vi "AlliGator Get Python Plugin API Version.vi"(8 "error in (no error)":errorcluster, 10 "Source":string, 11 "Script Header":string) -> (0 "error out":errorcluster, 1 "API Version":string, 3 "Script Header - Version":string)   [LabVIEW 2021, in "AlliGator Python Plugins.lvlib"]
uses:
  AlliGator Python Plugins.lvlib
panel:
  # "see the AlliGator License on the block diagram (Ctrl+E or Window:Show Block Diagram)"
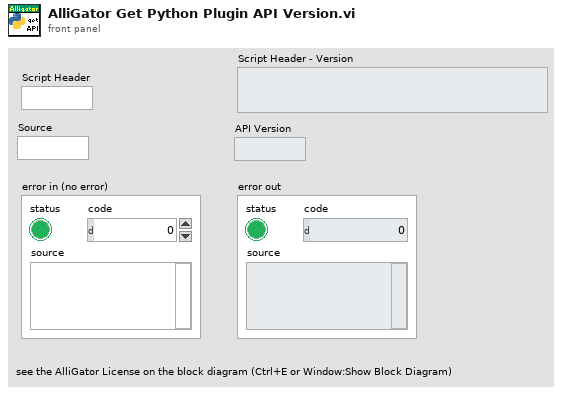
[diagram p1: front panel]
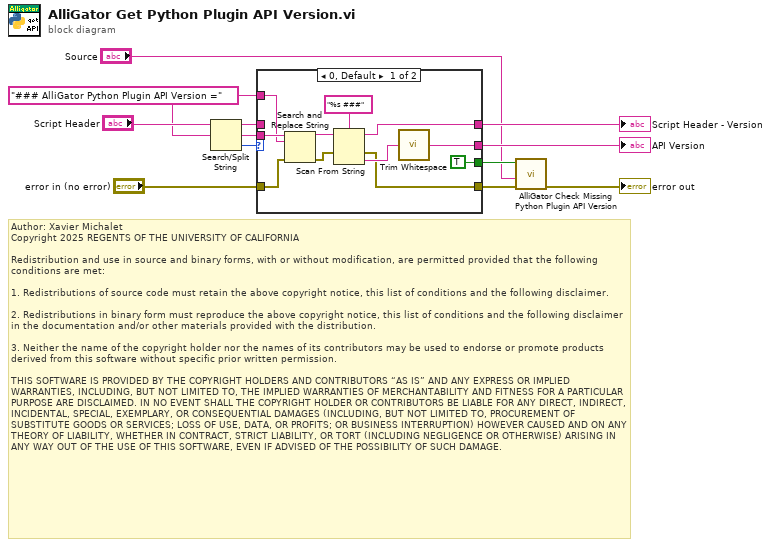
[diagram p0: block diagram]
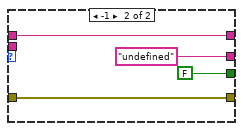
[diagram p2: hidden frame]
diagram:
  w9 = "### AlliGator Python Plugin API Version =" ("operators (none)")
  # "Author: Xavier Michalet\nCopyright 2025 REGENTS OF THE UNIVERSITY OF CALIFORNIA\n\nRedistribution and use in source and binary forms, with or without modification, are permitted provided that the following conditions are met:\n\n1. Redistributions of source code must retain the above copyright notice, this list of conditions and the following disclaimer.\n\n2. Redistributions in binary form must reproduce the above copyright notice, this list of conditions and the following disclaimer in the documentation and/or other materials provided with the distribution.\n\n3. Neither the name of the copyright holder nor the names of its contributors may be used to endorse or promote products derived from this software without specific prior written permission.\n\nTHIS SOFTWARE IS PROVIDED BY THE COPYRIGHT HOLDERS AND CONTRIBUTORS “AS IS” AND ANY EXPRESS OR IMPLIED WARRANTIES, INCLUDING, BUT NOT LIMITED TO, THE IMPLIED WARRANTIES OF MERCHANTABILITY AND FITNESS FOR A PARTICULAR PURPOSE ARE DISCLAIMED. IN NO EVENT SHALL THE COPYRIGHT HOLDER OR CONTRIBUTORS BE LIABLE FOR ANY DIRECT, INDIRECT, INCIDENTAL, SPECIAL, EXEMPLARY, OR CONSEQUENTIAL DAMAGES (INCLUDING, BUT NOT LIMITED TO, PROCUREMENT OF SUBSTITUTE GOODS OR SERVICES; LOSS OF USE, DATA, OR PROFITS; OR BUSINESS INTERRUPTION) HOWEVER CAUSED AND ON ANY THEORY OF LIABILITY, WHETHER IN CONTRACT, STRICT LIABILITY, OR TORT (INCLUDING NEGLIGENCE OR OTHERWISE) ARISING IN ANY WAY OUT OF THE USE OF THIS SOFTWARE, EVEN IF ADVISED OF THE POSSIBILITY OF SUCH DAMAGE."
  n1 = Search/Split String(string="Script Header", search string/char (-)=w9) -> (substring before match=w6:string, match + rest of string=w10:string, offset of match=w11:i32)  [unwired: 1 in]
  n2 = case shown="0, Default" w11 {
    tunnel: w10 -> [w23 _]
    tunnel: w9 -> [w22 _]
    tunnel: [w13 w26] -> w8
    tunnel: "error in (no error)" -> [w19 w27]
    tunnel: [w15 w27] -> w4
    tunnel: w6 -> [_ w26]
    tunnel: [w17 "undefined" ("API Version")] -> w5
    tunnel: [TRUE ("Function Name Found") FALSE ("Function Name Found")] -> w2
    frame 0, Default {
      n3 = Search and Replace String(input string=w23, search string=w22, error in=w19) -> (result string=w21:string, error out=w16:errorcluster)  [unwired: 5 in, 2 out]
      n4 = Scan From String(format string="%s ###", input string=w21, error in=w16) -> (remaining string=w13:string, error out=w15:errorcluster, output 1=w18:string)  [unwired: 2 in, 1 out]
      n5 = call <vilib>:"Trim Whitespace.vi"("string"=w18) -> ("trimmed string"=w17:string)  [unwired: 1 in]
    }
    frame -1 {
    }
  }
  "Script Header - Version" <- w8
  "API Version" <- w5
  n6 = call "AlliGator Check Missing Python Plugin API Version.vi"("error in (no error)"=w4, "Source"="Source", "Function Name Found"=w2) -> ("error out"=→"error out":errorcluster)  [unwired: 8 in]
